vi "Save to TDMS.vi"(7 "Exp Params in":T1={"Experiment Type"="2D Snapshot", "Experiment Name"="Experiment_1", "ExpPath"=path "E:/Data", "TSFrames"=1000, "TSfps"=1000, "ZTSFrames"=1000, "ZTSdt"=1, "Streaming"=FALSE, "Z Stack Settings"={"Start"=0.0, "Step Size"=0.1, "Finish"=1.0}, "total images"=1, "tdms ref"=refnum, "frame #"=0, "images per stack"=1, "total stacks"=1, "period"=1, "PI MVR Increment"=""} {"period" min=1; "total stacks" min=1; "images per stack" min=1; "total images" min=1; "Z Stack Settings"."Start" min=0.0 max=100.0 step=0.1; "Z Stack Settings"."Step Size" min=0.1 max=100.0 step=0.1; "Z Stack Settings"."Finish" min=0.0 max=100.0 step=0.1; "TSFrames" min=1 step=1; "ZTSdt" min=1 step=1; "ZTSFrames" min=2 step=1; "TSfps" min=1 max=1000 step=1}, 8 "error in (no error)":errorcluster, 9 "PI pos (um)":dbl, 10 "Timestamps (ns)":u64, 11 "pDataBuffer":u16[](array[numeric])) -> (0 "error out":errorcluster, 5 "Exp Params in out":T1={"Experiment Type"="2D Snapshot", "Experiment Name"="Experiment_1", "ExpPath"=path "E:/Data", "TSFrames"=1000, "TSfps"=1000, "ZTSFrames"=1000, "ZTSdt"=1, "Streaming"=FALSE, "Z Stack Settings"={"Start"=0.0, "Step Size"=0.1, "Finish"=1.0}, "total images"=1, "tdms ref"=refnum, "frame #"=0, "images per stack"=1, "total stacks"=1, "period"=1, "PI MVR Increment"=""} {"period" min=1; "total stacks" min=1; "images per stack" min=1; "total images" min=1; "Z Stack Settings"."Start" min=0.0 max=100.0 step=0.1; "Z Stack Settings"."Step Size" min=0.1 max=100.0 step=0.1; "Z Stack Settings"."Finish" min=0.0 max=100.0 step=0.1; "TSFrames" min=1 step=1; "ZTSdt" min=1 step=1; "ZTSFrames" min=2 step=1; "TSfps" min=1 max=1000 step=1})   [LabVIEW 2020]
uses:
  _Controls/Exp Params.ctl
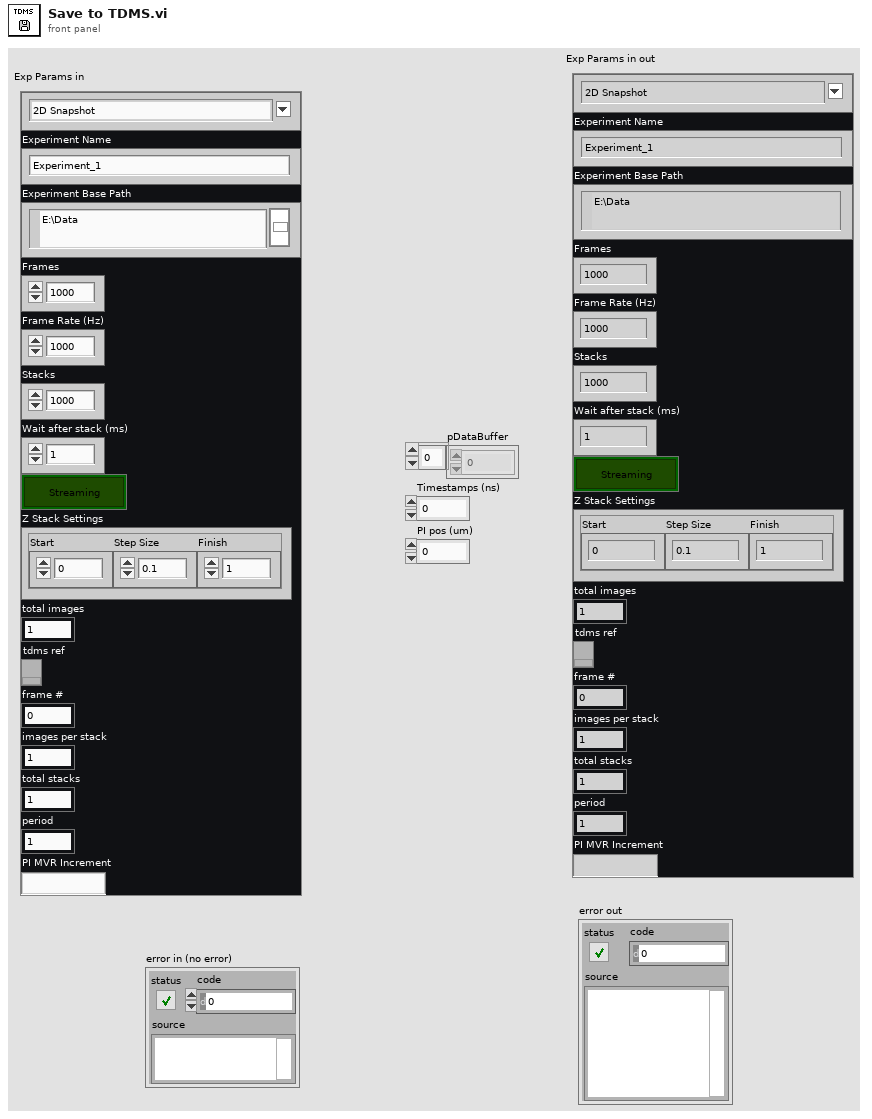
[diagram p1: front panel]
types:
  T1 = typedef "Exp Params.ctl" = cluster{"Experiment Type":string, "Experiment Name":string, "ExpPath":path, "TSFrames":i32, "TSfps":i32, "ZTSFrames":i32, "ZTSdt":i32, "Streaming":bool, "Z Stack Settings":cluster{"Start":dbl, "Step Size":dbl, "Finish":dbl}, "total images":i32, "tdms ref":refnum<k34>, "frame #":i64, "images per stack":i32, "total stacks":i32, "period":i32, "PI MVR Increment":string}
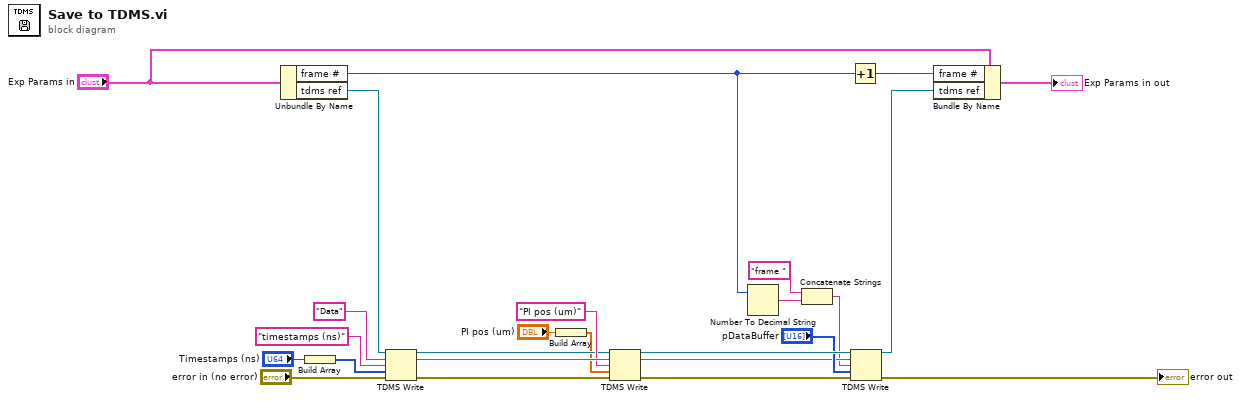
[diagram p0: block diagram]
diagram:
  n1 = Unbundle By Name("Exp Params in") -> ("frame #"=w4:i64, "tdms ref"=w25:refnum<k34>)
  n2 = Build Array("Timestamps (ns)") -> (w11:u64[])
  n3 = TDMS Write(0:w25, 5:"Data" ("group name in (Untitled)"), 7:"timestamps (ns)" ("group name in (Untitled)"), 9:w11, 11:"error in (no error)") -> (4:w18:refnum<k34>, 6:w21:string, 15:w19:errorcluster)  [unwired: 1 in, 1 out]
  n4 = Build Array("PI pos (um)") -> (w12:dbl[])
  n5 = TDMS Write(0:w18, 5:w21, 7:"PI pos (um)" ("group name in (Untitled)"), 9:w12, 11:w19) -> (4:w24:refnum<k34>, 6:w16:string, 15:w23:errorcluster)  [unwired: 1 in, 1 out]
  n6 = Number To Decimal String(number=w4) -> (decimal integer string=w6:string)  [unwired: 1 in]
  n7 = Concatenate Strings("frame ", w6) -> (w5:string)
  n8 = Increment(x=w4) -> (x+1=w3:i64)
  n9 = TDMS Write(0:w24, 5:w16, 7:w5, 9:"pDataBuffer", 11:w23) -> (4:w9:refnum<k34>, 15:→"error out":errorcluster)  [unwired: 1 in, 2 out]
  n10 = Bundle By Name(cluster="Exp Params in", "frame #"=w3, "tdms ref"=w9) -> (→"Exp Params in out":T1)
